vi "Set Frame User Events.vi"(8 "error in (no error)":errorcluster, 9 "Dynamic Events":T2(array[cluster]), 10 "Frame Index in":i32, 11 "Event Structure ref in":refnum<vi>) -> (0 "error out":errorcluster, 2 "Frame Index out":i32, 3 "Event Structure ref out":refnum<vi>)   [LabVIEW 2019, in "gRPC Scripting Tools.lvlib"]
uses:
  gRPC Scripting Tools.lvlib
  <vilib>/event_ctls.llb/lveventtype.ctl
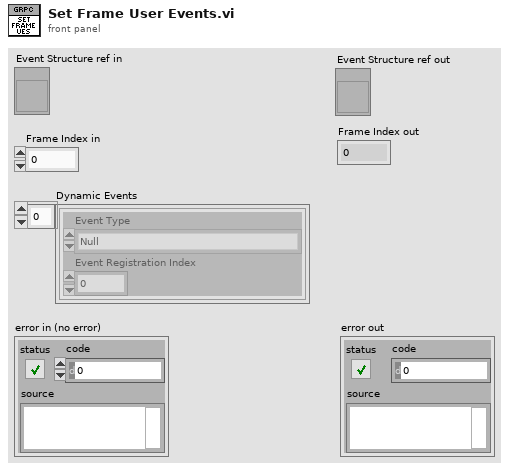
[diagram p1: front panel]
types:
  T1 = typedef "lveventtype.ctl" = enum32{"Null", "Timeout", "Annotation Menu Selection", "Annotation Menu Selection?", "App Instance Close", "App Instance Close?", "Autoscale Range Change", "Bookmark Info Change", "Cell Edit", "Cell Edit?", "Cursor Grab", "Cursor Grab?", "Cursor Menu Selection", "Cursor Menu Selection?", "Cursor Move", "Cursor Release", "Data Change", "Direction Change", "Display State Change", "Drag Ended", "Drag Enter", "Drag Leave", "Drag Over", "Drag Source Update", "Drag Starting", "Drag Starting?", "Drop", "Exec State Change", "Key Down", "Key Down?", "Key Repeat", "Key Repeat?", "Key Up", "Listbox Double Click", "Menu Activation?", "Menu Selection (App)", "Menu Selection? (App)", "Menu Selection (User)", "Mouse Down", "Mouse Down?", "Mouse Enter", "Mouse Leave", "Mouse Move", "Mouse Up", "Mouse Wheel", "NI Security User Change (App)", "Pane Size", "Panel Close", "Panel Close?", "Panel Resize", "Plot Attribute Change", "Scale Range Change", "Shortcut Menu Activation?", "Shortcut Menu Selection (App)", "Shortcut Menu Selection? (App)", "Shortcut Menu Selection (User)", "Tree Double Click", "Tree Drag", "Tree Drag?", "Tree Drop", "Tree Drop?", "Tree Item Close", "Tree Item Close?", "Tree Item Open", "Tree Item Open?", "User Event", "Value Change"}
  T2 = cluster{"Event Type":T1, "Event Registration Index":i32}[]
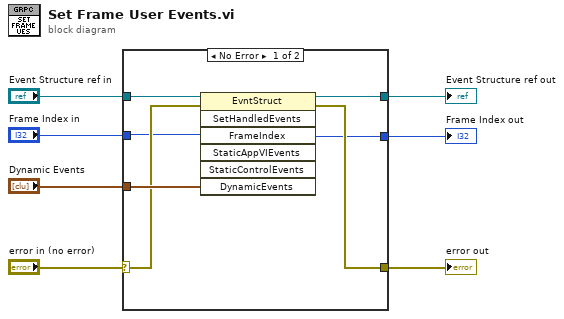
[diagram p0: block diagram]
diagram:
  n1 = case shown="No Error" "error in (no error)" {
    selector: "error in (no error)" -> [w9 w15]
    tunnel: "Frame Index in" -> [w8 w14]
    tunnel: [w13 w15] -> w6
    tunnel: "Dynamic Events" -> [w12 _]
    tunnel: "Event Structure ref in" -> [w11 w16]
    tunnel: [w10 w16] -> w3
    tunnel: [w8 w14] -> w1
    frame No Error {
      n2 = invoke class="EvntStruct" method="SetHandledEvents"(reference=w11, error in=w9, "FrameIndex"=w8, "DynamicEvents"=w12) -> (reference out=w10:refnum<vi>, error out=w13:errorcluster)  [unwired: 3 in, 5 out]
    }
    frame Error {
    }
  }
  "error out" <- w6
  "Event Structure ref out" <- w3
  "Frame Index out" <- w1
